vi "Configure Multi Eval Meas List Segment ACLR.vi"(0 "VISA resource name":refnum<visa-resource-name>, 1 "Enable (Off)":bool, 2 "UTRA 2 (Off)":bool, 5 "Instance (1)":T1=1, 7 "Segment (1)":i32=1, 9 "Statistics (20)":i32=20, 11 "error in (no error)":errorcluster, 12 "UTRA 1 (Off)":bool, 13 "NR (Off)":bool) -> (4 "VISA resource name out":refnum<visa-resource-name>, 15 "error out":errorcluster)   [LabVIEW 2020, in "Rohde&Schwarz CMWXP NR FR1 Measurement.lvlib"]
doc: "Defines settings for ACLR measurements in list mode for segment <no>.\n\nAttribute:\nRSCMWXPNRFR1M_ATTR_MULTI_EVAL_MEAS_LIST_SEGMENT_ACLR\n\nRemote-control command:\nCONFigure:NRSub:MEAS<i>:MEValuation:LIST:SEGMent<no>:ACLR"
uses:
  <instrlib>/Rohde&Schwarz CMWXP NR FR1 Measurement/Rohde&Schwarz CMWXP NR FR1 Measurement.lvlib
  <instrlib>/Rohde&Schwarz CMWXP NR FR1 Measurement/Private/_Instance.ctl
  <instrlib>/Rohde&Schwarz CMWXP NR FR1 Measurement/Private/rsidr_core.llb/rsidr_core.lvlib
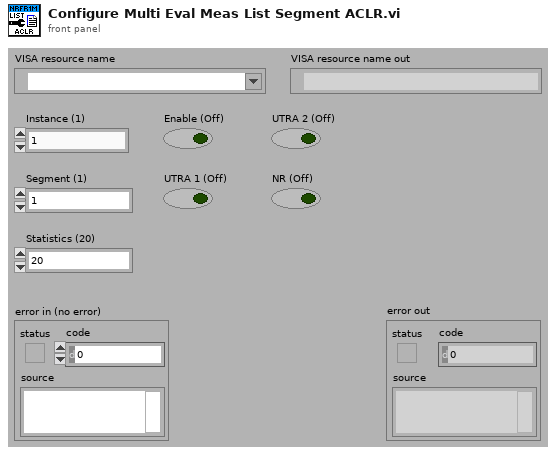
[diagram p1: front panel]
types:
  T1 = typedef "Rohde&Schwarz CMWXP NR FR1 Measurement.lvlib/_Instance.ctl" = i32
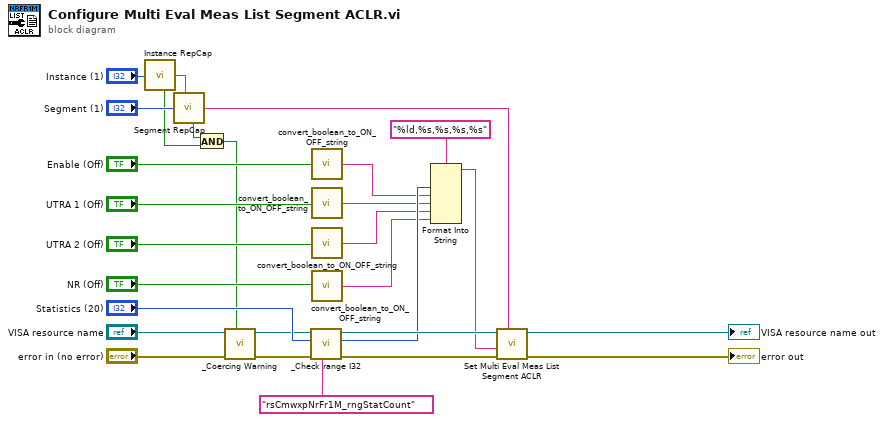
[diagram p0: block diagram]
diagram:
  n1 = call <instrlib>:"Instance RepCap.vi"("Instance In"="Instance (1)") -> ("In Range?"=w7:bool, "RepCap Identifier Out"=w26:string)  [unwired: 1 in]
  n2 = call <instrlib>:"Segment RepCap.vi"("Segment In"="Segment (1)", "RepCap String In (\"\")"=w26) -> ("In Range?"=w6:bool, "RepCap Identifier Out"=w25:string)
  n3 = And(x=w6, y=w7) -> (x .and. y?=w1:bool)
  n4 = call <instrlib>:"_Coercing Warning.vi"("In Range?"=w1, "error in (no error)"="error in (no error)", "VISA resource name"="VISA resource name") -> ("error out"=w3:errorcluster, "VISA resource name out"=w2:refnum<visa-resource-name>)  [unwired: 7 in]
  n5 = call <instrlib>:"_Check range I32.vi"("Range Table Identifier"="rsCmwxpNrFr1M_rngStatCount", "error in (no error)"=w3, "I32 Value In"="Statistics (20)", "VISA resource name"=w2) -> ("error out"=w23:errorcluster, "I32 Value Out"=w17:i32, "VISA resource name out"=w20:refnum<visa-resource-name>)  [unwired: 5 in]
  n6 = call <instrlib>:"convert_boolean_to_ON_OFF_string.vi"("boolean value in"="Enable (Off)") -> ("string value out"=w12:string)  [unwired: 4 in]
  n7 = call <instrlib>:"convert_boolean_to_ON_OFF_string.vi"("boolean value in"="UTRA 1 (Off)") -> ("string value out"=w11:string)  [unwired: 4 in]
  n8 = call <instrlib>:"convert_boolean_to_ON_OFF_string.vi"("boolean value in"="UTRA 2 (Off)") -> ("string value out"=w10:string)  [unwired: 4 in]
  n9 = call <instrlib>:"convert_boolean_to_ON_OFF_string.vi"("boolean value in"="NR (Off)") -> ("string value out"=w9:string)  [unwired: 4 in]
  n10 = Format Into String(format string="%ld,%s,%s,%s,%s", w17, w12, w11, w10, w9) -> (resulting string=w8:string)  [unwired: 2 in, 1 out]
  n11 = call "Set Multi Eval Meas List Segment ACLR"("Repeated Capabilities"=w25, "error in (no error)"=w23, "Multi Eval Meas List Segment ACLR ()"=w8, "instrument handle"=w20) -> ("error out"=→"error out":errorcluster, "instrument handle out"=→"VISA resource name out":refnum<visa-resource-name>)  [unwired: 6 in]
